vi "test_webcam.vi"() -> ()   [LabVIEW 2019]
uses:
  <vilib>/userDefined/High Color/IMAQdx.ctl
panel:
  in  "camera cfg":cluster{"Port":T1, "Camera file":path}={"Port"="cam2", "Camera file"=path "C:/AGV/Config/camera/C920_1024X576_30fps.icd"}
  out "Image":T2(plugin-control)
  in  "dt":u32=30
  out "숫자형":i32
  in  "정지":bool
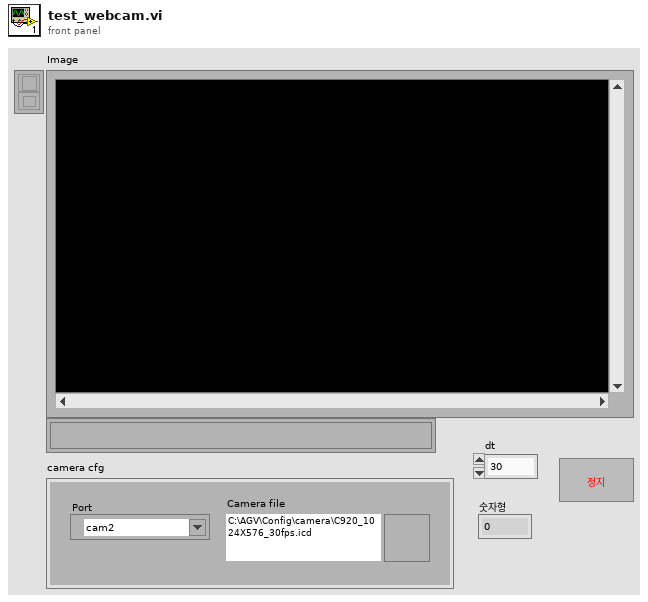
[diagram p1: front panel]
types:
  T1 = typedef "IMAQdx.ctl" = refnum<k21>
  T2 = typedef "IMAQ Image.ctl" = refnum<image>
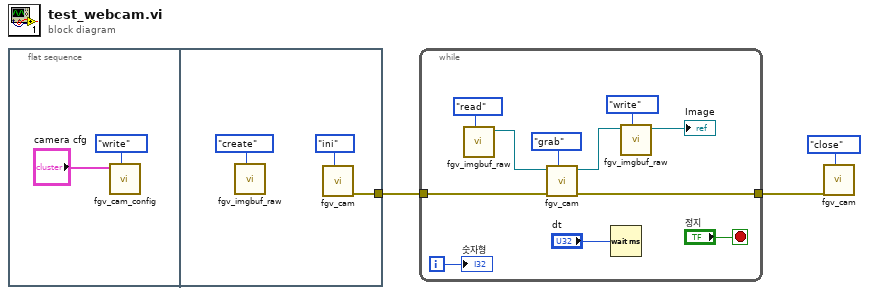
[diagram p0: block diagram]
diagram:
  n1 = flat-sequence {
    tunnel: [w7] -> w3
    frame #0 {
      n2 = call "fgv_cam_config.vi"("cmd"=enum16{"read", "write"}."write", "camera cfg"="camera cfg") -> ()  [unwired: 9 in, 1 out]
    }
    frame #1 {
      n3 = call "fgv_imgbuf_raw.vi"("cmd"=enum16{"create", "close", "write", "read"}."create") -> ()  [unwired: 9 in, 2 out]
      n4 = call "fgv_cam.vi"("cmd"=enum16{"ini", "grab", "close", "read"}."ini") -> ("error out"=w7:errorcluster)  [unwired: 8 in, 2 out]
    }
  }
  n5 = while {
    tunnel: w3 -> [w18]
    tunnel: [w15] -> w2
    i -> [w14]
    stop <- "정지" stop-if-true
    n6 = call "fgv_imgbuf_raw.vi"("cmd"=enum16{"create", "close", "write", "read"}."read") -> ("Image"=w16:T2)  [unwired: 9 in, 1 out]
    n7 = call "fgv_cam.vi"("cmd"=enum16{"ini", "grab", "close", "read"}."grab", "error in"=w18, "Image In"=w16) -> ("error out"=w15:errorcluster, "Image Out"=w11:T2)  [unwired: 6 in, 1 out]
    n8 = Wait (ms)(milliseconds to wait="dt") -> ()  [unwired: 1 out]
    n9 = call "fgv_imgbuf_raw.vi"("cmd"=enum16{"create", "close", "write", "read"}."write", "raw Image in"=w11) -> ("Image"=→"Image":T2)  [unwired: 8 in, 1 out]
    "숫자형" <- w14
  }
  n10 = call "fgv_cam.vi"("cmd"=enum16{"ini", "grab", "close", "read"}."close", "error in"=w2) -> ()  [unwired: 7 in, 3 out]
